vi "GenerateIniFile.vi"() -> ()   [LabVIEW 2017, in "Server.lvlib"]
uses:
  Server.lvlib
  TypeDefs/ServerINI.ctl
  SubLibs/Oracle/OracleData.ctl
  SubLibs/Oracle/Oracle.lvlib
panel:
  in  "ServerINI":T1={"TrackQueues?"=TRUE, "ClientTimeout (s)"=30, "LogPath"=path "", "ErrorsToIgnore"=[], "OracleData"={"DBname"="", "User"="", "Password"=""}}
  out "error out":errorcluster
  in  "INI Path":path
  in  "Defaul INI-Directory?":bool=TRUE
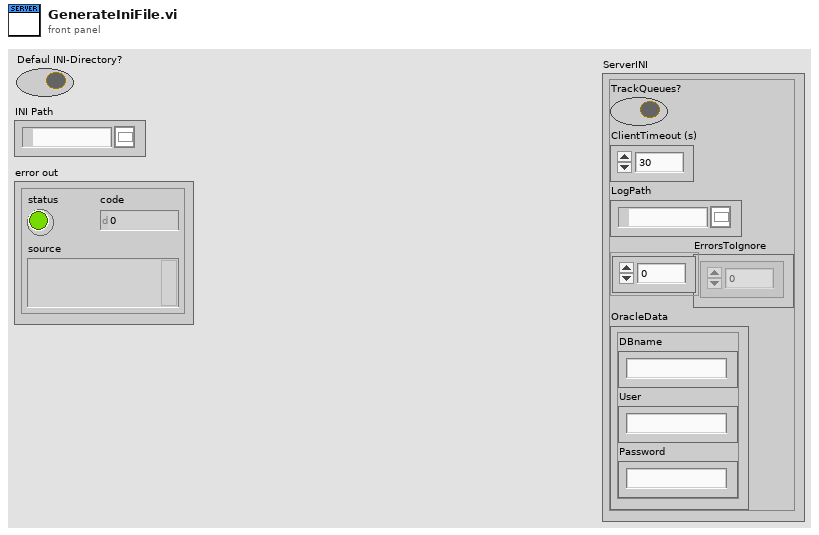
[diagram p1: front panel]
types:
  T1 = typedef "Server.lvlib/ServerINI.ctl" = cluster{"TrackQueues?":bool, "ClientTimeout (s)":u32, "LogPath":path, "ErrorsToIgnore":i32[], "OracleData":T2}
  T2 = typedef "Server.lvlib/Oracle.lvlib/OracleData.ctl" = cluster{"DBname":string, "User":string, "Password":string}
  T3 = enum16{"open", "replace", "create", "open or create", "replace or create", "replace or create with confirmation"}
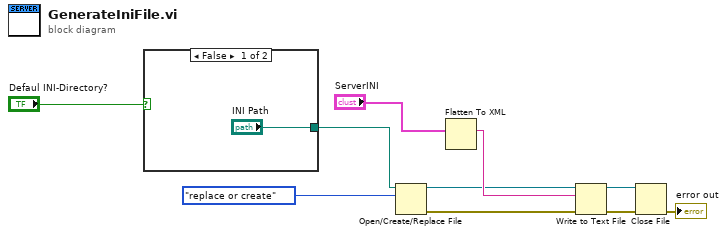
[diagram p0: block diagram]
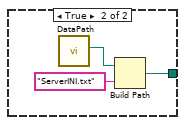
[diagram p2: hidden frame]
diagram:
  n1 = case shown="False" "Defaul INI-Directory?" {
    tunnel: ["INI Path" w12] -> w10
    frame False {
    }
    frame True {
      n2 = call "DataPath.vi"() -> ("DataDirectory"=w13:path)  [unwired: 11 in]
      n3 = Build Path(base path=w13, name or relative path="ServerINI.txt") -> (appended path=w12:path)
    }
  }
  n4 = Open/Create/Replace File(file path (use dialog)=w10, operation (0:open)=T3."replace or create") -> (refnum out=w6:refnum<file>, error out=w5:errorcluster)  [unwired: 4 in, 1 out]
  n5 = Flatten To XML(anything="ServerINI") -> (xml string=w7:string)
  n6 = Write to Text File(file (use dialog)=w6, text=w7, error in=w5) -> (refnum out=w4:refnum<file>, error out=w3:errorcluster)  [unwired: 1 in, 1 out]
  n7 = Close File(refnum=w4, error in=w3) -> (error out=→"error out":errorcluster)  [unwired: 1 out]
